vi "简单工厂模式客户端.vi"() -> ()   [LabVIEW 2011]
panel:
  out "运算结果":dbl
  in  "输入B":dbl
  in  "输入A":dbl
  in  "运算":T1
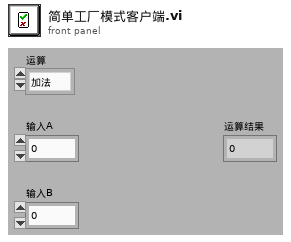
[diagram p1: front panel]
types:
  T1 = typedef "运算工厂.lvclass/运算方法.ctl" = enum16{"加法", "减法", "乘法", "平方和"}
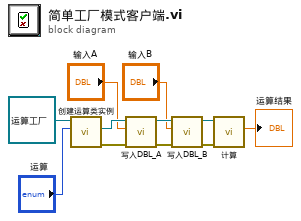
[diagram p0: block diagram]
diagram:
  n1 = call "创建运算类实例.vi"("运算"="运算", "运算工厂 输入"=refnum<class "运算工厂.lvclass"> refnum ("运算工厂.lvclass")) -> ("error out"=w7:errorcluster, "运算类.lvclass"=w10:refnum<class "运算类.lvclass">)  [unwired: 7 in, 1 out]
  n2 = call "写入DBL_A.vi"("error in (no error)"=w7, "DBL_A"="输入A", "运算类输入"=w10) -> ("error out"=w6:errorcluster, "运算类输出"=w9:refnum<class "运算类.lvclass">)  [unwired: 7 in]
  n3 = call "写入DBL_B.vi"("error in (no error)"=w6, "DBL_B"="输入B", "运算类输入"=w9) -> ("error out"=w3:errorcluster, "运算类输出"=w4:refnum<class "运算类.lvclass">)  [unwired: 7 in]
  n4 = call-dynamic "计算.vi"("error in (no error)"=w3, "运算类 输入"=w4) -> ("结果"=→"运算结果":dbl)  [unwired: 7 in, 2 out]
